vi "Close XWPF Writer.vi"(8 "error in (no error)":errorcluster, 11 "xwpfWriter in":refnum<class "xwpfWriter.lvclass">) -> (0 "error out":errorcluster, 3 "xwpfWriter out":refnum<class "xwpfWriter.lvclass">)   [LabVIEW 2017, in "xwpfWriter.lvclass"]
doc: "Closes the XWPFDocument and the XWPFExtractor references."
uses:
  xwpfWriter.lvclass
  xwpfWriter.lvclass/xwpfWriter.ctl
  Support/File Stream/File Stream.lvlib
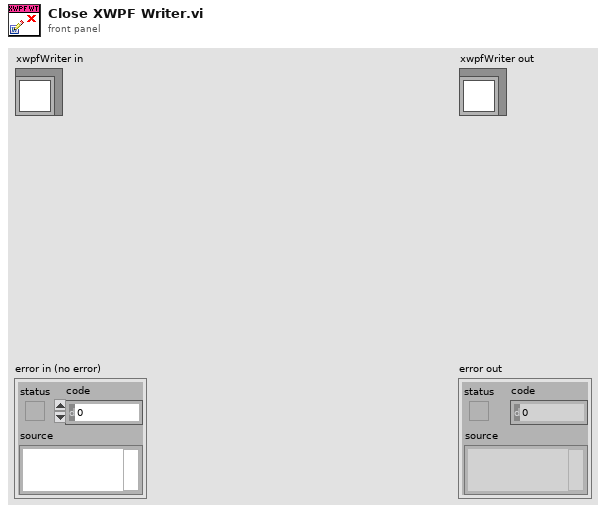
[diagram p1: front panel]
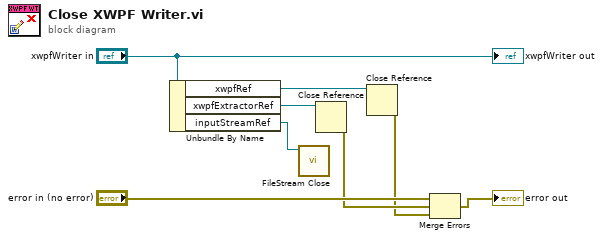
[diagram p0: block diagram]
diagram:
  n1 = Unbundle By Name("xwpfWriter in") -> ("xwpfRef"=w3:refnum<k24>, "xwpfExtractorRef"=w5:refnum<k24>, "inputStreamRef"=w1:refnum<k24>)
  n2 = call "FileStream Close.vi"("reference"=w1) -> ()  [unwired: 10 in, 1 out]
  n3 = Close Reference(reference=w5) -> (error out=w4:errorcluster)  [unwired: 1 in]
  n4 = Close Reference(reference=w3) -> (error out=w2:errorcluster)  [unwired: 1 in]
  n5 = Merge Errors("error in (no error)", w4, w2) -> (→"error out":errorcluster)
  "xwpfWriter out" <- "xwpfWriter in"
